vi "FRIC_navX_Internal_SPI_ProcessingLoop.vi"(7 "Device Number":T1, 9 "Clock Rate (Hz)":dbl=2000000.0 format="%_6f", 10 "SPI Bus":T2=enum."SPI MXP", 11 "Update Rate (4Hz-200Hz)":u8=50 min=4 max=200) -> ()   [LabVIEW 2015]
doc: "This navX VI handles the reading/writing for the navX. All of the good stuff is in here.\nTHIS VI SHOULD NOT BE CALLED BY THE USER!"
uses:
  <vilib>/Rock Robotics/SystemInterfaces/spilib/spi_bus.ctl
  _TypeDefs/FRIC_navX_DeviceNumbersTypeDef.ctl
  _TypeDefs/FRIC_navX_I2C Process Loop TypeDef.ctl
  _TypeDefs/FRIC_navX_ProcessingLoopStatesTypeDef_I2C.ctl
  _TypeDefs/Z900_navX_DeviceTypeDef.ctl
  _TypeDefs/Z900_navX_ProtocolTypeDef.ctl
  _TypeDefs/Z900_navX_NotifyPacketTypeDef.ctl
  _TypeDefs/Z900_navX_ActionTypeDef.ctl
  _TypeDefs/Z900_navX_SerialStreamTypeDef.ctl
  <vilib>/Rock Robotics/SystemInterfaces/i2clib/i2c_bus.ctl
  _TypeDefs/Z900_navX_IntegrationControlRegisters.ctl
  <vilib>/Rock Robotics/WPI/SPI/WPI_SPIDevRef.ctl
  _NI WPI Serial USB/WPI_SerialPort_USB.ctl
  <vilib>/Rock Robotics/WPI/SerialPort/WPI_SerialPortRef.ctl
  _TypeDefs/Flags/Z900_navX_Flags_CapabilityTypeDef.ctl
  _TypeDefs/Z900_navX_DeviceRegisters.ctl
  <vilib>/Rock Robotics/SystemInterfaces/Utilities/FPGA_UtilitiesRead LocalTime.vi
  _NI WPI Serial USB/_NI WPI Serial USB.lvlib
panel:
  out "Loop Time (ms)":dbl
  out "Connected":bool
  in  "Halt":bool
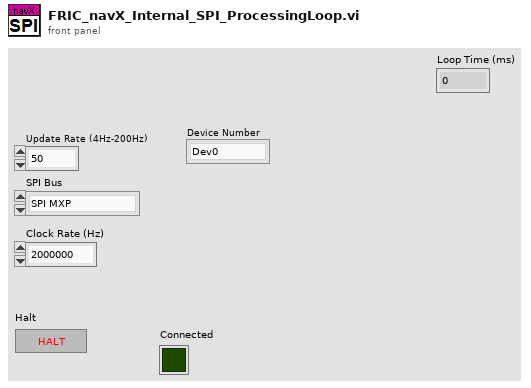
[diagram p1: front panel]
types:
  T1 = typedef "FRIC_navX_DeviceNumbersTypeDef.ctl" = enum16{"Dev0", "Dev1", "Dev2", "Dev3", "Dev4", "Dev5", "Dev6", "Dev7", "Dev8", "Dev9", "Dev10"}
  T2 = typedef "spi_bus.ctl" = enum16{"SPI On-Board, CS0", "SPI On-Board, CS1", "SPI On-Board, CS2", "SPI On-Board, CS3", "SPI MXP", "Invalid"}
  T3 = typedef "FRIC_navX_I2C Process Loop TypeDef.ctl" = cluster{"State Array":T4[], "error":errorcluster, "FPGA Cluster":cluster{"Last Valid FPGA Time":dbl, "Error Count":i32, "Initialized":bool}, "Device Info":T5, "I2CDevRef":cluster{"DevStatus":errorcluster, "Device Address":u8, "Handle":i32, "I2C Bus":T7}, "Registry":u8[], "Command Array":T8[], "Connected?":bool, "navX Device Memory Size":i32, "notification":T9, "Memory Size Set":bool, "SPIDevRef":T12, "navX Serial Open":cluster{"Serial Port":T13, "Stream Type":T11}, "SerialPortRef":T14, "Serial Read Buffer":string, "Serial Write Buffer":string[], "Device Number":T1, "navX SPI Open":cluster{"SPI Bus":T2, "Clock Rate (Hz)":dbl}}
  T4 = typedef "FRIC_navX_ProcessingLoopStatesTypeDef_I2C.ctl" = enum16{"Process", "INI", "Check Packets Valid", "Close", "Flush Serial", "Generate Command", "Last Packet Valid", "Open", "Read", "Reset Serial", "Set Termination Char", "Update AE", "Wait", "Write", "Exit"}
  T5 = typedef "Z900_navX_DeviceTypeDef.ctl" = cluster{"Interface":cluster{"Protocol":T6, "Update Rate (4Hz-200Hz)":u8, "navX Open TypeDef":variant}, "Notify Packet":refnum<notifier>, "Loop VI Refnum":refnum<vi>, "Ready to Close Occurrence Refnum":refnum<k4>, "Name":string}
  T6 = typedef "Z900_navX_ProtocolTypeDef.ctl" = enum16{"SERIAL", "I2C", "SPI"}
  T7 = typedef "i2c_bus.ctl" = enum16{"I2C On-Board", "I2C MXP", "Invalid"}
  T8 = typedef "Z900_navX_IntegrationControlRegisters.ctl" = u8
  T9 = typedef "Z900_navX_NotifyPacketTypeDef.ctl" = cluster{"navX Action":T10, "Data":variant, "Stream Type":T11}
  T10 = typedef "Z900_navX_ActionTypeDef.ctl" = enum16{"None", "Halt", "Normal Read", "Update Serial Protocol", "Update Rate Htz", "Zero-Yaw", "Zero-Displacement", "Zero-Velocity"}
  T11 = typedef "Z900_navX_SerialStreamTypeDef.ctl" = enum16{"YRPH", "Quaterinons", "Gyro/Raw", "AHRS", "AHRSAndPositioning"}
  T12 = typedef "WPI_SPIDevRef.ctl" = cluster{"DevStatus":errorcluster, "Handle":i32, "SPI Bus":T2}
  T13 = typedef "_NI WPI Serial USB.lvlib/WPI_SerialPort_USB.ctl" = enum16{"Onboard RS-232", "MXP TTL", "USB"}
  T14 = typedef "WPI_SerialPortRef.ctl" = cluster{"DevStatus":errorcluster, "Serial Port Name":refnum<visa-resource-name>}
  T15 = typedef "Z900_navX_DeviceRegisters.ctl" = u8
  T16 = typedef "Z900_navX_Flags_CapabilityTypeDef.ctl" = u16
  T17 = cluster{"Last Valid FPGA Time":dbl, "Error Count":i32, "Initialized":bool}
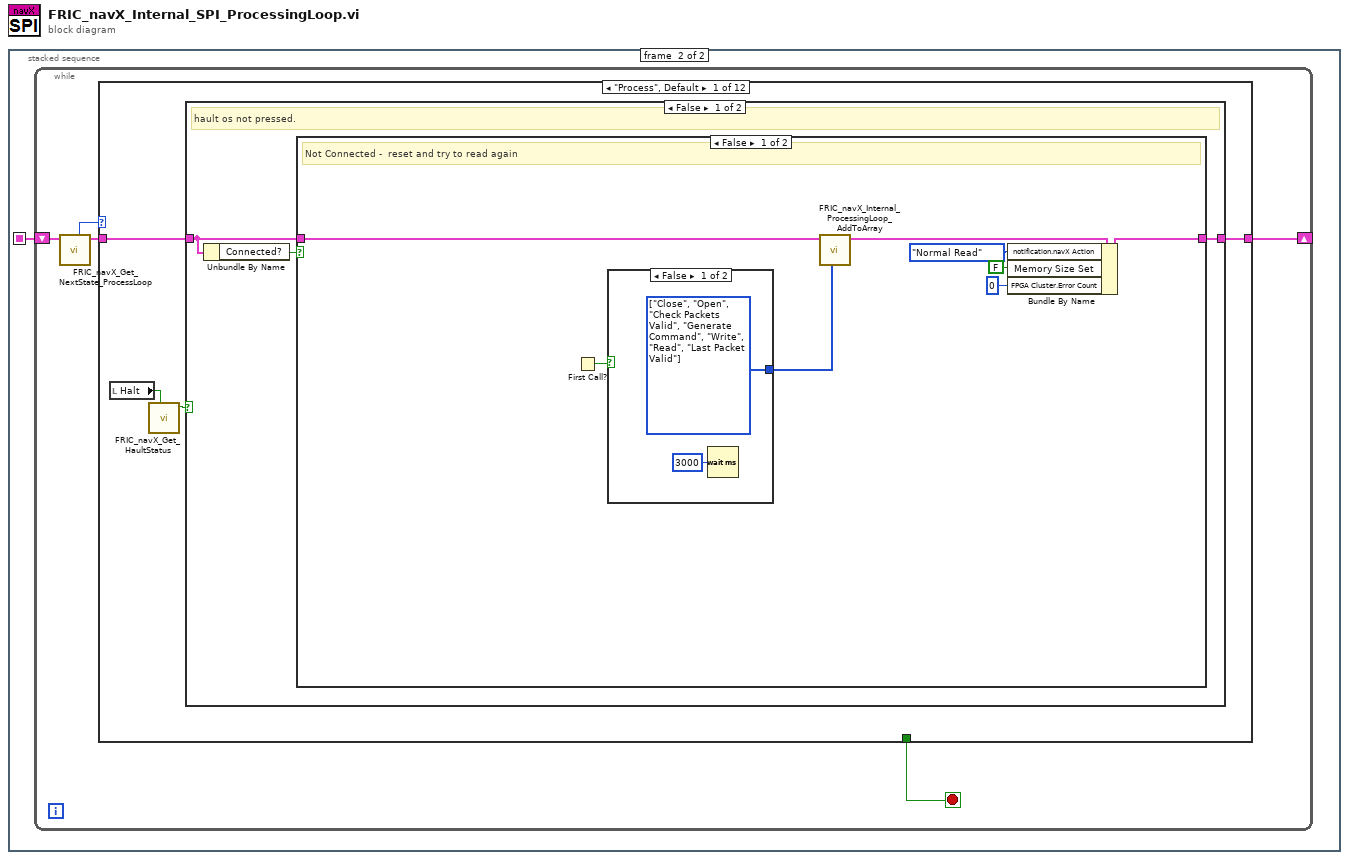
[diagram p0: block diagram]
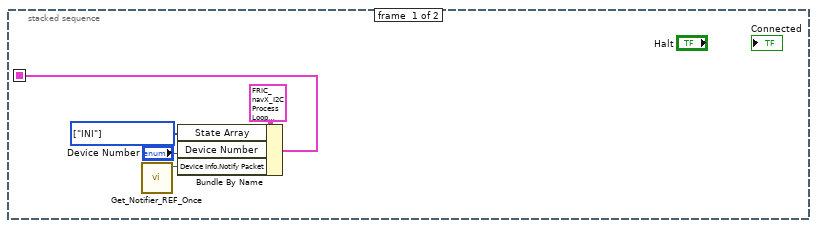
[diagram p2: hidden frame]
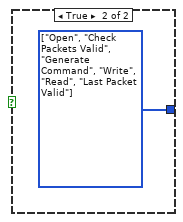
[diagram p3: hidden frame]
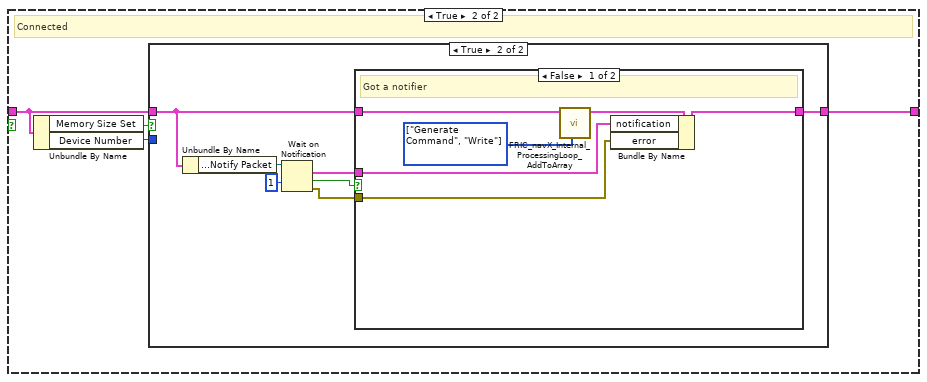
[diagram p4: hidden frame]
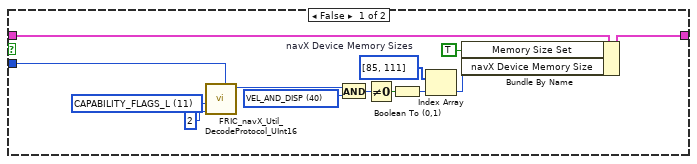
[diagram p5: hidden frame]
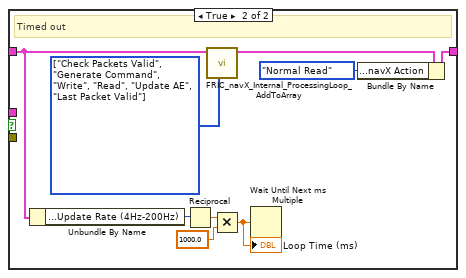
[diagram p6: hidden frame]
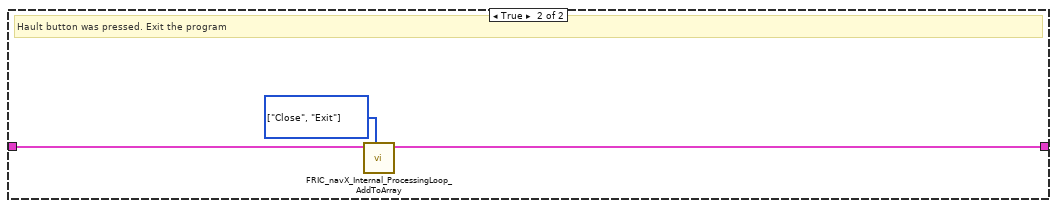
[diagram p7: hidden frame]
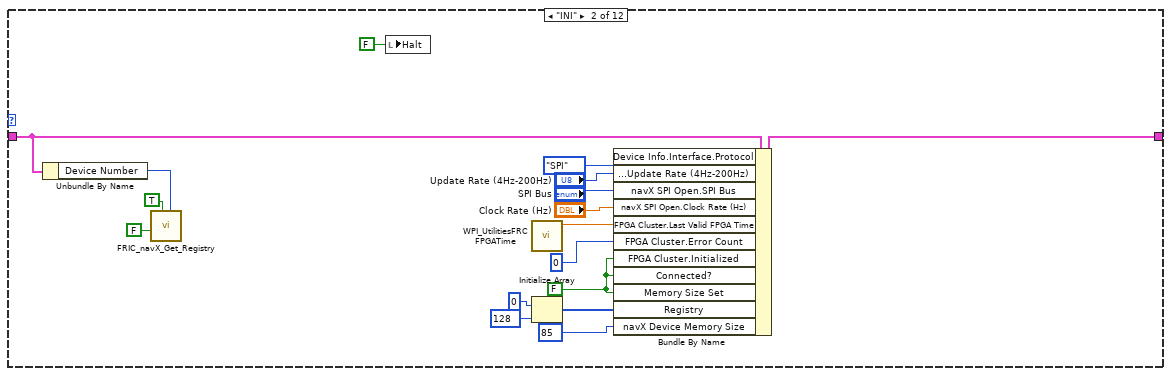
[diagram p8: hidden frame]
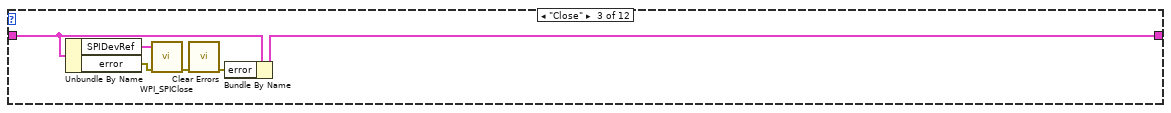
[diagram p9: hidden frame]
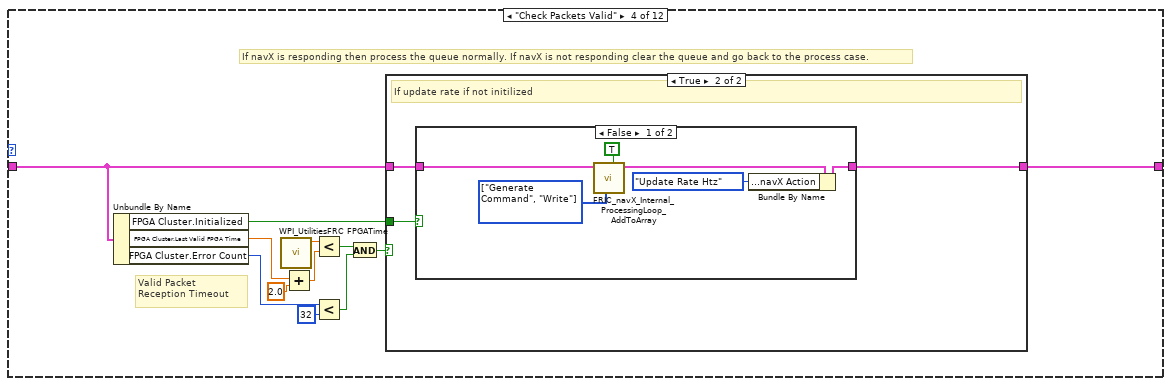
[diagram p10: hidden frame]
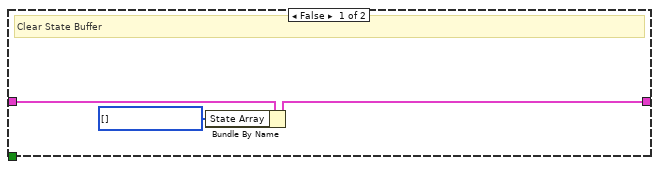
[diagram p11: hidden frame]
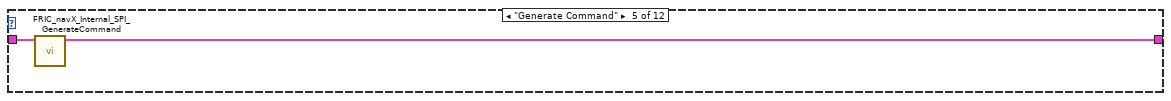
[diagram p13: hidden frame]
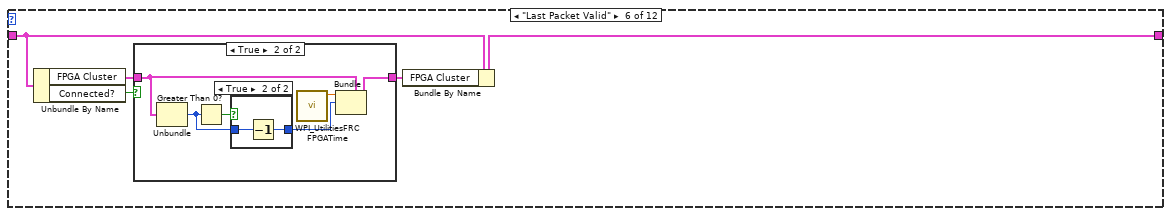
[diagram p14: hidden frame]
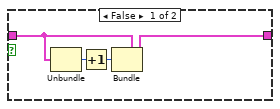
[diagram p15: hidden frame]
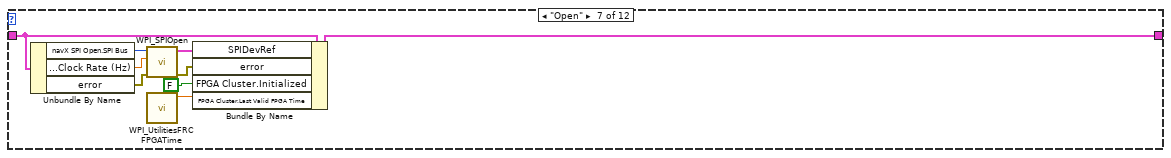
[diagram p17: hidden frame]
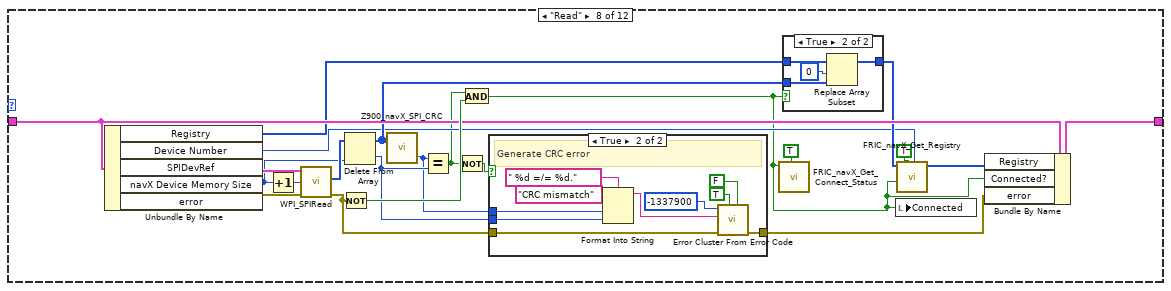
[diagram p18: hidden frame]
diagram:
  n1 = stacked-sequence {
    seq-local: [w5 _] -> [_ w6]
    frame #0 {
      w3 = T4[] [enum."INI"] items=["Process", "INI", "Check Packets Valid", "Close", "Flush Serial", "Generate Command", "Last Packet Valid", "Open", "Read", "Reset Serial", "Set Termination Char", "Update AE", "Wait", "Write", "Exit"] ("State Array")
      n2 = call "Get_Notifier_REF_Once.vi"() -> ("notifier ref out"=w1:refnum<notifier>)  [unwired: 10 in, 1 out]
      n3 = Bundle By Name(cluster=T3 {"State Array"=[enum."INI", enum."Open"], "error"={"status"=FALSE, "code"=0, "source"=""}, "FPGA Cluster"={"Last Valid FPGA Time"=0.0, "Error Count"=0, "Initialized"=FALSE}, "Device Info"={"Interface"={"Protocol"=enum."SERIAL", "Update Rate (4Hz-200Hz)"=4, "navX Open TypeDef"=variant}, "Notify Packet"=refnum, "Loop VI Refnum"=refnum, "Ready to Close Occurrence Refnum"=refnum, "Name"=""}, "I2CDevRef"={"DevStatus"={"status"=FALSE, "code"=0, "source"=""}, "Device Address"=0, "Handle"=0, "I2C Bus"=enum."Invalid"}, "Registry"=[], "Command Array"=[214, 32], "Connected?"=FALSE, "navX Device Memory Size"=85, "notification"={"navX Action"=enum."None", "Data"=variant, "Stream Type"=enum."YRPH"}, "Memory Size Set"=FALSE, "SPIDevRef"={"DevStatus"={"status"=FALSE, "code"=0, "source"=""}, "Handle"=0, "SPI Bus"=enum."SPI On-Board, CS0"}, "navX Serial Open"={"Serial Port"=enum."Onboard RS-232", "Stream Type"=enum."YRPH"}, "SerialPortRef"={"DevStatus"={"status"=FALSE, "code"=0, "source"=""}, "Serial Port Name"=""}, "Serial Read Buffer"="", "Serial Write Buffer"=[], "Device Number"=enum."Dev0", "navX SPI Open"={"SPI Bus"=enum."SPI MXP", "Clock Rate (Hz)"=500000.0}} ("I2C Process Loop TypeDef"), "State Array"=w3, "Device Number"="Device Number", "Device Info.Notify Packet"=w1) -> (w5:T3)
    }
    frame #1 {
      n4 = while {
        shift-right: [w7] -> _
        shift-left: w6 -> [w10]
        stop <- w11 stop-if-true
        n5 = call "FRIC_navX_Get_NextState_ProcessLoop.vi"("I2C Process Loop TypeDef (in)"=w10) -> ("I2C Process Loop TypeDef (out)"=w9:T3, "Current State"=w8:T4)  [unwired: 9 in]
        n6 = case shown="\"Process\", Default" w8 {
          tunnel: [_ _ _ _ _ _ _ _ _ _ TRUE _] -> w11
          tunnel: w9 -> [w14 w75 w94 w98 w121 w125 w148 w168 w188 w194 w197 w205]
          tunnel: [w15 w81 w93 w99 w120 w124 w147 w167 w188 w195 w197 w205] -> w7
          frame "Process", Default {
            n7 = local read "Halt"() -> (w13:bool)
            n8 = call "FRIC_navX_Get_HaultStatus.vi"("Update"=w13) -> ("Hault"=w12:bool)  [unwired: 10 in]
            n9 = case shown="False" w12 {
              tunnel: [w18 w70] -> w15
              tunnel: w14 -> [w16 w71]
              frame False {
                # "hault os not pressed."
                n10 = Unbundle By Name(w16) -> ("Connected?"=w17:bool)
                n11 = case shown="False" w17 {
                  tunnel: w16 -> [w26 w32]
                  tunnel: [w23 w33] -> w18
                  frame False {
                    # "Not Connected -  reset and try to read again"
                    n12 = First Call?() -> (First Call?: T/F=w19:bool)
                    n13 = case shown="False" w19 {
                      tunnel: [w28 w29] -> w25
                      frame False {
                        w28 = T4[] [enum."Close", enum."Open", enum."Check Packets Valid", enum."Generate Command", enum."Write", enum."Read", enum."Last Packet Valid"] items=["Process", "INI", "Check Packets Valid", "Close", "Flush Serial", "Generate Command", "Last Packet Valid", "Open", "Read", "Reset Serial", "Set Termination Char", "Update AE", "Wait", "Write", "Exit"]
                        n14 = Wait (ms)(milliseconds to wait=u32 3000) -> ()  [unwired: 1 out]
                      }
                      frame True {
                        w29 = T4[] [enum."Open", enum."Check Packets Valid", enum."Generate Command", enum."Write", enum."Read", enum."Last Packet Valid"] items=["Process", "INI", "Check Packets Valid", "Close", "Flush Serial", "Generate Command", "Last Packet Valid", "Open", "Read", "Reset Serial", "Set Termination Char", "Update AE", "Wait", "Write", "Exit"]
                      }
                    }
                    n15 = call "FRIC_navX_Internal_ProcessingLoop_AddToArray.vi"("States Array"=w25, "I2C Process Loop TypeDef (in)"=w26) -> ("I2C Process Loop TypeDef (out)"=w24:T3)  [unwired: 9 in]
                    n16 = Bundle By Name(cluster=w24, "notification.navX Action"=Z900_navX_ActionTypeDef."Normal Read", "Memory Size Set"=FALSE, "FPGA Cluster.Error Count"=0) -> (w23:T3)
                  }
                  frame True {
                    # "Connected"
                    n17 = Unbundle By Name(w32) -> ("Memory Size Set"=w31:bool, "Device Number"=w30:T1)
                    n18 = case shown="True" w31 {
                      tunnel: [w45 w51] -> w33
                      tunnel: w32 -> [w46 w48]
                      tunnel: w30 -> [w34 _]
                      frame False {
                        w44 = T15 11 items=["WHOAMI"=0, "HW_REV"=1, "FW_VER_MAJOR"=2, "FW_VER_MINOR"=3, "UPDATE_RATE_HZ"=4, "ACCEL_FSR_G"=5, "GYRO_FSR_DPS"=6, "OP_STATUS"=8, "CAL_STATUS"=9, "SELFTEST_STATUS"=10, "CAPABILITY_FLAGS_L"=11, "CAPABILITY_FLAGS_H"=12, "SENSOR_STATUS"=16, "TIMESTAMP"=18, "YAW"=22, "ROLL"=24, "PITCH"=26, "HEADING"=28, "FUSED_HEADING"=30, "ALTITUDE_I"=32, "ALTITUDE_D"=34, "LINERA_ACC_X"=36, "LINERA_ACC_Y"=38, "LINERA_ACC_Z"=40, "QUAT_W"=42, "QUAT_X"=44, "QUAT_Y"=46, "QUAT_Z"=48, "MPU_TEMP_C"=50, "GYRO_X"=52, "GYRO_Y"=54, "GYRO_Z"=56, "ACC_X"=58, "ACC_Y"=60, "ACC_Z"=62, "MAG_X"=64, "MAG_Y"=66, "MAG_Z"=68, "PRESSURE_I"=70, "PRESSURE_D"=72, "PRESSURE_TEMP"=74, "YAW_OFFSET"=76, "QUAT_OFFSET_W"=78, "QUAT_OFFSET_X"=80, "QUAT_OFFSET_Y"=82, "QUAT_OFFSET_Z"=84, "INTEGRATION_CONTROL"=86, "VELOCITY_X"=88, "VELOCITY_Y"=92, "VELOCITY_Z"=96, "DISPLACMENT_X"=100, "DISPLACMENT_Y"=104, "DISPLACEMENT_Z"=108] ("Device Register")
                        w39 = T16 40 items=["OMNIMOUNT"=4, "OMNIMOUNT_CONFIG_MASK"=38, "VEL_AND_DISP"=40, "YAW_RESET"=80] ("Capability Flag")
                        w40 = i32[] [85, 111]  # navX Device Memory Sizes
                        n19 = call "FRIC_navX_Util_DecodeProtocol_UInt16.vi"("Device Number"=w34, "length"=2, "Device Register"=w44) -> ("Value"=w37:u16)  [unwired: 8 in]
                        n20 = And(x=w37, y=w39) -> (x .and. y?=w38:T16)
                        n21 = Not Equal To 0?(x=w38) -> (x != 0?=w41:bool)
                        n22 = Boolean To (0,1)(Boolean=w41) -> (0, 1=w42:i16)
                        n23 = Index Array(array=w40, index=w42) -> (element=w35:i32)
                        n24 = Bundle By Name(cluster=w46, "Memory Size Set"=TRUE, "navX Device Memory Size"=w35) -> (w45:T3)
                      }
                      frame True {
                        n25 = Unbundle By Name(w48) -> ("Device Info.Notify Packet"=w53:refnum<notifier>)
                        n26 = Wait on Notification(notifier=w53, timeout in ms (-1)=1) -> (notification=w50:T9, timed out?=w47:bool, error out=w49:errorcluster)  [unwired: 2 in, 1 out]
                        n27 = case shown="False" w47 {
                          tunnel: w48 -> [w59 w67]
                          tunnel: [w58 w65] -> w51
                          tunnel: w50 -> [w57 _]
                          tunnel: w49 -> [w54 _]
                          frame False {
                            w55 = T4[] [enum."Generate Command", enum."Write"] items=["Process", "INI", "Check Packets Valid", "Close", "Flush Serial", "Generate Command", "Last Packet Valid", "Open", "Read", "Reset Serial", "Set Termination Char", "Update AE", "Wait", "Write", "Exit"] ("States Array")
                            # "Got a notifier"
                            n28 = call "FRIC_navX_Internal_ProcessingLoop_AddToArray.vi"("States Array"=w55, "I2C Process Loop TypeDef (in)"=w59) -> ("I2C Process Loop TypeDef (out)"=w56:T3)  [unwired: 9 in]
                            n29 = Bundle By Name(cluster=w56, "notification"=w57, "error"=w54) -> (w58:T3)
                          }
                          frame True {
                            w68 = T4[] [enum."Check Packets Valid", enum."Generate Command", enum."Write", enum."Read", enum."Update AE", enum."Last Packet Valid"] items=["Process", "INI", "Check Packets Valid", "Close", "Flush Serial", "Generate Command", "Last Packet Valid", "Open", "Read", "Reset Serial", "Set Termination Char", "Update AE", "Wait", "Write", "Exit"]
                            # "Timed out"
                            n30 = Unbundle By Name(w67) -> ("Device Info.Interface.Update Rate (4Hz-200Hz)"=w63:u8)
                            n31 = Reciprocal(x=w63) -> (1/x=w62:dbl)
                            n32 = call "FRIC_navX_Internal_ProcessingLoop_AddToArray.vi"("States Array"=w68, "I2C Process Loop TypeDef (in)"=w67) -> ("I2C Process Loop TypeDef (out)"=w66:T3)  [unwired: 9 in]
                            n33 = Multiply(x=w62, y=1000.0) -> (x*y=w60:dbl)
                            "Loop Time (ms)" <- w60
                            n34 = Wait Until Next ms Multiple(millisecond multiple=w60) -> ()  [unwired: 1 out]
                            n35 = Bundle By Name(cluster=w66, "notification.navX Action"=Z900_navX_ActionTypeDef."Normal Read") -> (w65:T3)
                          }
                        }
                      }
                    }
                  }
                }
              }
              frame True {
                w69 = T4[] [enum."Close", enum."Exit"] items=["Process", "INI", "Check Packets Valid", "Close", "Flush Serial", "Generate Command", "Last Packet Valid", "Open", "Read", "Reset Serial", "Set Termination Char", "Update AE", "Wait", "Write", "Exit"] ("States Array")
                # "Hault button was pressed. Exit the program"
                n36 = call "FRIC_navX_Internal_ProcessingLoop_AddToArray.vi"("States Array"=w69, "I2C Process Loop TypeDef (in)"=w71) -> ("I2C Process Loop TypeDef (out)"=w70:T3)  [unwired: 9 in]
              }
            }
          }
          frame "INI" {
            w79 = FALSE ("Initialized")
            n37 = Unbundle By Name(w75) -> ("Device Number"=w74:T1)
            n38 = call "FRIC_navX_Get_Registry.vi"("Device Number"=w74, "Update"=TRUE, "Connected?"=FALSE) -> ()  [unwired: 7 in, 2 out]
            n39 = local write "Halt"(FALSE ("Halt")) -> ()
            n40 = call <vilib>:"WPI_UtilitiesFRC FPGATime.vi"() -> ("FPGA Time"=w83:dbl)  [unwired: 10 in, 1 out]
            n41 = Initialize Array(u8 0 ("Received Data"), 128 ("hex")) -> (w77:u8[])
            n42 = Bundle By Name(cluster=w75, "Device Info.Interface.Protocol"=Z900_navX_ProtocolTypeDef."SPI" ("Protocol"), "Device Info.Interface.Update Rate (4Hz-200Hz)"="Update Rate (4Hz-200Hz)", "navX SPI Open.SPI Bus"="SPI Bus", "navX SPI Open.Clock Rate (Hz)"="Clock Rate (Hz)", "FPGA Cluster.Last Valid FPGA Time"=w83, "FPGA Cluster.Error Count"=0 ("Error Count"), "FPGA Cluster.Initialized"=w79, "Connected?"=w79, "Memory Size Set"=w79, "Registry"=w77, "navX Device Memory Size"=85 ("hex")) -> (w81:T3)
          }
          frame "Close" {
            n43 = Unbundle By Name(w94) -> ("SPIDevRef"=w92:T12, "error"=w91:errorcluster)
            n44 = call <vilib>:"WPI_SPIClose.vi"("error in (no error)"=w91, "SPIDevRef"=w92) -> ("error out"=w90:errorcluster)  [unwired: 9 in]
            n45 = call <vilib>:"Clear Errors.vi"("error in (no error)"=w90) -> ("error out"=w89:errorcluster)  [unwired: 5 in, 1 out]
            n46 = Bundle By Name(cluster=w94, "error"=w89) -> (w93:T3)
          }
          frame "Check Packets Valid" {
            # "If navX is responding then process the queue normally. If navX is not responding clear the queue and go back to the process case."
            # "Valid Packet Reception Timeout"
            n47 = Unbundle By Name(w98) -> ("FPGA Cluster.Initialized"=w96:bool, "FPGA Cluster.Last Valid FPGA Time"=w97:dbl, "FPGA Cluster.Error Count"=w95:i32)
            n48 = call <vilib>:"WPI_UtilitiesFRC FPGATime.vi"() -> ("FPGA Time"=w104:dbl)  [unwired: 10 in, 1 out]
            n49 = Add(x=w97, y=2.0) -> (x+y=w105:dbl)
            n50 = Less?(x=w104, y=w105) -> (x < y?=w102:bool)
            n51 = Less?(x=w95, y=32) -> (x < y?=w101:bool)
            n52 = And(x=w102, y=w101) -> (x .and. y?=w100:bool)
            n53 = case shown="True" w100 {
              tunnel: w98 -> [w109 w112]
              tunnel: [w108 w111] -> w99
              tunnel: w96 -> [_ w110]
              frame False {
                w107 = T4[] [] items=["Process", "INI", "Check Packets Valid", "Close", "Flush Serial", "Generate Command", "Last Packet Valid", "Open", "Read", "Reset Serial", "Set Termination Char", "Update AE", "Wait", "Write", "Exit"] ("f")
                # "Clear State Buffer"
                n54 = Bundle By Name(cluster=w109, "State Array"=w107) -> (w108:T3)
              }
              frame True {
                # "If update rate if not initilized"
                n55 = case shown="False" w110 {
                  tunnel: w112 -> [w117 w119]
                  tunnel: [w115 w119] -> w111
                  frame False {
                    w113 = T4[] [enum."Generate Command", enum."Write"] items=["Process", "INI", "Check Packets Valid", "Close", "Flush Serial", "Generate Command", "Last Packet Valid", "Open", "Read", "Reset Serial", "Set Termination Char", "Update AE", "Wait", "Write", "Exit"] ("f")
                    n56 = call "FRIC_navX_Internal_ProcessingLoop_AddToArray.vi"("Add to beginning"=TRUE, "States Array"=w113, "I2C Process Loop TypeDef (in)"=w117) -> ("I2C Process Loop TypeDef (out)"=w116:T3)  [unwired: 8 in]
                    n57 = Bundle By Name(cluster=w116, "notification.navX Action"=Z900_navX_ActionTypeDef."Update Rate Htz") -> (w115:T3)
                  }
                  frame True {
                  }
                }
              }
            }
          }
          frame "Generate Command" {
            n58 = call "FRIC_navX_Internal_SPI_GenerateCommand.vi"("I2C Process Loop TypeDef (in)"=w121) -> ("I2C Process Loop TypeDef (out)"=w120:T3)  [unwired: 10 in]
          }
          frame "Last Packet Valid" {
            n59 = Unbundle By Name(w125) -> ("FPGA Cluster"=w126:T17, "Connected?"=w122:bool)
            n60 = case shown="True" w122 {
              tunnel: [w129 w136] -> w123
              tunnel: w126 -> [w128 w132]
              frame False {
                n61 = Unbundle(w128) -> ("Error Count"=w127:i32)  [unwired: 2 out]
                n62 = Increment(x=w127) -> (x+1=w130:i32)
                n63 = Bundle(cluster=w128, "Error Count"=w130) -> (w129:T17)  [unwired: 2 in]
              }
              frame True {
                n64 = Unbundle(w132) -> ("Error Count"=w131:i32)  [unwired: 2 out]
                n65 = Greater Than 0?(x=w131) -> (x > 0?=w134:bool)
                n66 = case shown="True" w134 {
                  tunnel: [w137 w139] -> w133
                  tunnel: w131 -> [w137 w138]
                  frame False {
                  }
                  frame True {
                    n67 = Decrement(x=w138) -> (x-1=w139:i32)
                  }
                }
                n68 = call <vilib>:"WPI_UtilitiesFRC FPGATime.vi"() -> ("FPGA Time"=w135:dbl)  [unwired: 10 in, 1 out]
                n69 = Bundle(cluster=w132, "Last Valid FPGA Time"=w135, "Error Count"=w133) -> (w136:T17)  [unwired: 1 in]
              }
            }
            n70 = Bundle By Name(cluster=w125, "FPGA Cluster"=w123) -> (w124:T3)
          }
          frame "Open" {
            n71 = Unbundle By Name(w148) -> ("navX SPI Open.SPI Bus"=w141:T2, "navX SPI Open.Clock Rate (Hz)"=w140:dbl, "error"=w142:errorcluster)
            n72 = call <vilib>:"WPI_SPIOpen.vi"("error in"=w142, "Clock Rate (Hz)"=w140, "SPI Bus"=w141) -> ("error out"=w144:errorcluster, "SPIDevRef"=w145:T12)  [unwired: 7 in]
            n73 = call <vilib>:"WPI_UtilitiesFRC FPGATime.vi"() -> ("FPGA Time"=w143:dbl)  [unwired: 10 in, 1 out]
            n74 = Bundle By Name(cluster=w148, "SPIDevRef"=w145, "error"=w144, "FPGA Cluster.Initialized"=FALSE ("Initialized"), "FPGA Cluster.Last Valid FPGA Time"=w143) -> (w147:T3)
          }
          frame "Read" {
            n75 = Unbundle By Name(w168) -> ("Registry"=w165:u8[], "Device Number"=w154:T1, "SPIDevRef"=w164:T12, "navX Device Memory Size"=w157:i32, "error"=w163:errorcluster)
            n76 = Increment(x=w157) -> (x+1=w156:i32)
            n77 = call <vilib>:"WPI_SPIRead.vi"("error in (no error)"=w163, "Num to Read"=w156, "SPIDevRef"=w164) -> ("error out"=w160:errorcluster, "Received Data"=w162:u8[])  [unwired: 6 in, 1 out]
            n78 = Not(x=w160) -> (.not. x?=w169:bool)
            n79 = Delete From Array(array=w162, index=w157) -> (deleted portion=w158:u8, array with subset deleted=w155:u8[])  [unwired: 1 in]
            n80 = call "Z900_navX_SPI_CRC.vi"("Message"=w155) -> ("CRC"=w153:u8)  [unwired: 1 out]
            n81 = Equal?(x=w153, y=w158) -> (x = y?=w151:bool)
            n82 = Not(x=w151) -> (.not. x?=w152:bool)
            n83 = And(x=w151, y=w169) -> (x .and. y?=w149:bool)
            n84 = case shown="True" w152 {
              tunnel: w153 -> [_ w179]
              tunnel: w158 -> [_ w178]
              tunnel: w160 -> [w171 w175]
              tunnel: [w171 w174] -> w159
              frame False {
              }
              frame True {
                # "Generate CRC error"
                n85 = Format Into String(format string=" %d =/= %d.", initial string="CRC mismatch", w179, w178) -> (resulting string=w176:string)  [unwired: 1 in, 1 out]
                n86 = call <vilib>:"Error Cluster From Error Code.vi"("is warning? (False)"=FALSE, "show call chain? (False)"=TRUE, "error in (no error)"=w175, "error message (\"\")"=w176, "error code (0)"=-1337900 ("code")) -> ("error out"=w174:errorcluster)  [unwired: 4 in]
              }
            }
            n87 = call "FRIC_navX_Get_Connect_Status.vi"("Update"=TRUE, "Connected"=w149) -> ()  [unwired: 9 in, 1 out]
            n88 = case shown="True" w149 {
              tunnel: w165 -> [w182 w186]
              tunnel: [w182 w185] -> w161
              tunnel: w155 -> [_ w184]
              frame False {
              }
              frame True {
                n89 = Replace Array Subset(array=w186, new element=w184, index=u8 0 ("hex")) -> (w185:u8[])
              }
            }
            n90 = local write "Connected"(w149) -> ()
            n91 = call "FRIC_navX_Get_Registry.vi"("Device Number"=w154, "Update"=TRUE, "Connected?"=w149, "Registry (in)"=w161) -> ("Registry (out)"=w166:u8[])  [unwired: 6 in, 1 out]
            n92 = Bundle By Name(cluster=w168, "Registry"=w166, "Connected?"=w149, "error"=w159) -> (w167:T3)
          }
          frame "Wait" {
            n93 = Wait (ms)(milliseconds to wait=u32 1) -> ()  [unwired: 1 out]
          }
          frame "Write" {
            n94 = Unbundle By Name(w194) -> ("SPIDevRef"=w193:T12, "Command Array"=w192:T8[], "I2CDevRef.DevStatus"=w191:errorcluster)
            n95 = call <vilib>:"WPI_SPIWrite.vi"("error in (no error)"=w191, "Data To Send"=w192, "SPIDevRef"=w193) -> ("error out"=w190:errorcluster, "SPIDevRef"=w189:T12)  [unwired: 6 in, 1 out]
            n96 = Bundle By Name(cluster=w194, "SPIDevRef"=w189, "error"=w190) -> (w195:T3)
          }
          frame "Exit" {
            n97 = Unbundle By Name(w197) -> ("Device Info"=w196:T5)
            n98 = in-place {
              in-place-border: [TRUE] -> w199
              in-place-border: w196 -> [w200]
              # "Set Occurence of Close"
              n99 = Unbundle By Name(w200) -> ("Ready to Close Occurrence Refnum"=w202:refnum<k4>)
              n100 = local write "Halt"(FALSE ("Halt")) -> ()
              n101 = Set Occurrence(w202) -> ()
            }
            n102 = Stop(stop? (T)=w199) -> ()
          }
          frame "Update AE" {
            n103 = Unbundle By Name(w205) -> ("Device Number"=w204:T1)
            n104 = call "FRIC_navX_Internal_ProcessingLoop_UpdateAE.vi"("Device Number"=w204) -> ()  [unwired: 5 in, 10 out]
          }
        }
      }
    }
  }
